vi "init_LiCor (moose's).vi"() -> ()   [LabVIEW 2010]
uses:
  <vilib>/Instr/_visa.llb/VISA Configure Serial Port (Instr).vi
panel:
  in  "String 3":string="(RS232(Poll Now))\\n "
  in  "String 2":string="(Display(BackLt\\s1))\\n "
  in  "String":string="(RS232(Sources (\"CO2B um/m\" \"H2OB mm/m\"  \"Integral\" \"Peak\" \"P kPa\" \"T C\" ))) "
  in  "Text_out 2":string
  in  "Text_out 1":string
  out "Text 2":string
  out "Text1":string
  out "VISA resource name 2":refnum<visa-resource-name>="ASRL2::INSTR"
  out "error out":errorcluster
  in  "init?":bool=TRUE
  in  "VISA resource name":refnum<visa-resource-name>="COM11"
  in  "error in":errorcluster
  in  "Quit?":bool=TRUE
  in  "Port Configuration":T1={"baud rate (9600)"=9600, "data bits (8)"=8, "parity (0:none)"=enum."None", "stop bits (10: 1 bit)"=10, "flow control (0:none)"=3, "timeout (10sec)"=10000, "termination char\n(0xA = '\\n' = LF) "=10, "Enable Termination\nChar (T)"=TRUE} {"termination char\n(0xA = '\\n' = LF)" format="%.0x"; "flow control (0:none)" items=["None", "XON/XOFF", "RTS/CTS", "XON/XOFF & RTS/CTS", "DTR/DSR", "XON/XOFF & DTR/DSR"]; "stop bits (10: 1 bit)" items=["1.0"=10, "1.5"=15, "2.0"=20]; "data bits (8)" min=5 max=8 step=1}
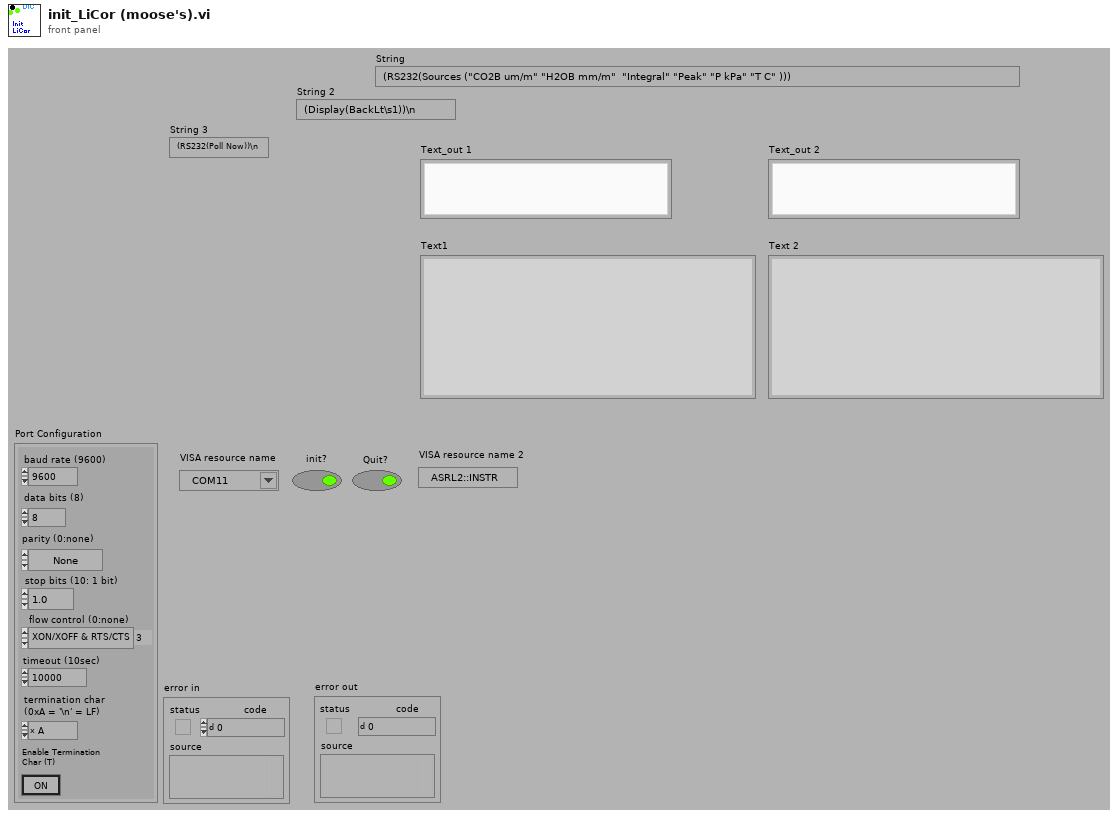
[diagram p1: front panel]
types:
  T1 = cluster{"baud rate (9600)":u32, "data bits (8)":u16, "parity (0:none)":enum16{"None", "Odd", "Even", "Mark", "Space"}, "stop bits (10: 1 bit)":u16, "flow control (0:none)":u16, "timeout (10sec)":u32, "termination char\n(0xA = '\\n' = LF) ":u8, "Enable Termination\nChar (T)":bool}
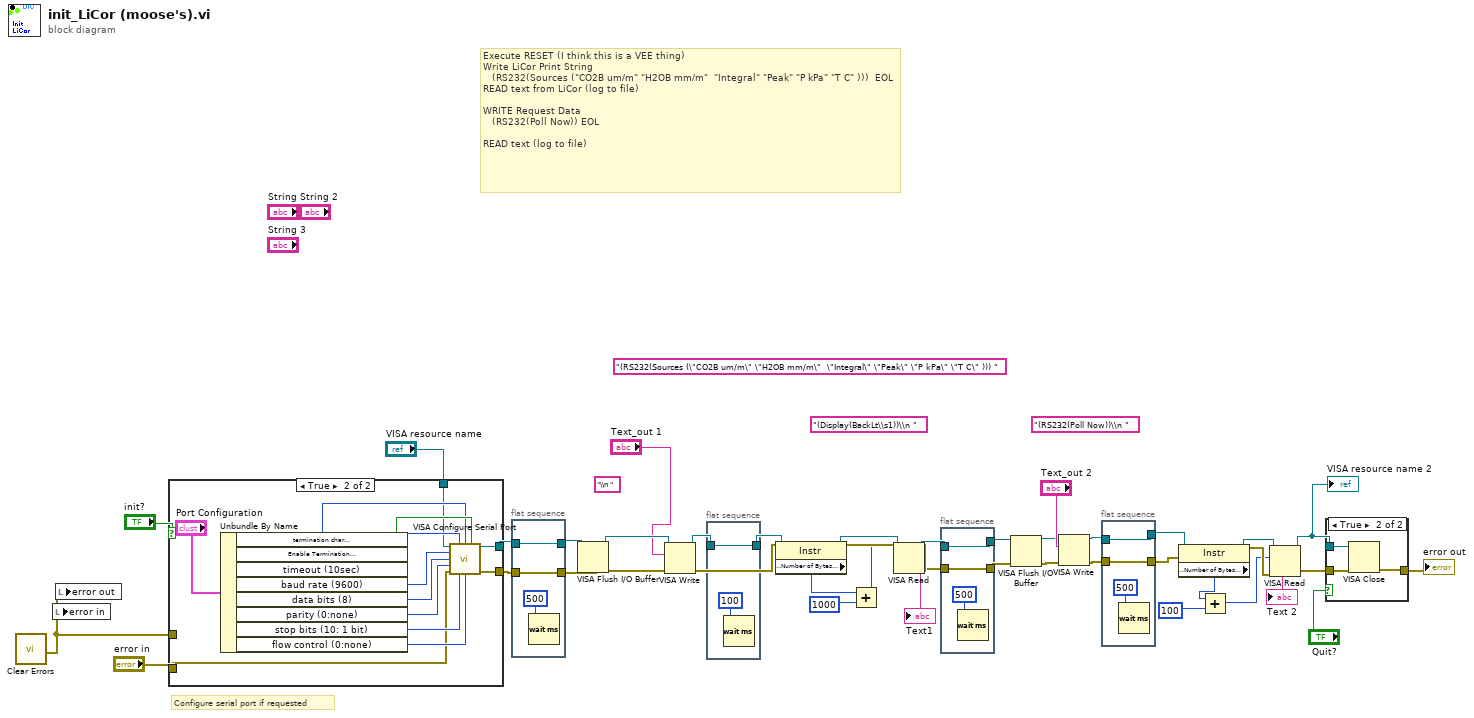
[diagram p0: block diagram]
diagram:
  (unwired) "\\n "
  (unwired) "(Display(BackLt\\s1))\\n "
  (unwired) "(RS232(Poll Now))\\n "
  (unwired) "(RS232(Sources (\"CO2B um/m\" \"H2OB mm/m\"  \"Integral\" \"Peak\" \"P kPa\" \"T C\" ))) "
  # "Configure serial port if requested"
  # "Execute RESET (I think this is a VEE thing)\nWrite LiCor Print String \n   (RS232(Sources (\"CO2B um/m\" \"H2OB mm/m\"  \"Integral\" \"Peak\" \"P kPa\" \"T C\" )))  EOL\nREAD text from LiCor (log to file)\n\nWRITE Request Data\n   (RS232(Poll Now)) EOL\n\nREAD text (log to file)"
  n1 = call <vilib>:"Clear Errors.vi"() -> ("error out"=w2:errorcluster)  [unwired: 7 in]
  n2 = local write "error in"(w2) -> ()
  n3 = local write "error out"(w2) -> ()
  n4 = case shown="True" "init?" {
    tunnel: [w42 w47] -> w21
    tunnel: [w43 w46] -> w19
    tunnel: "error in" -> [w43 w45]
    tunnel: "VISA resource name" -> [w42 w44]
    tunnel: w2 -> [_ _]
    frame False {
    }
    frame True {
      n5 = Unbundle By Name("Port Configuration") -> ("termination char\n(0xA = '\\n' = LF)"=w48:u8, "Enable Termination\nChar (T)"=w49:bool, "timeout (10sec)"=w50:u32, "baud rate (9600)"=w55:u32, "data bits (8)"=w54:u16, "parity (0:none)"=w53:enum16{"None", "Odd", "Even", "Mark", "Space"}, "stop bits (10: 1 bit)"=w52:u16, "flow control (0:none)"=w51:u16)
      n6 = call-poly "VISA Configure Serial Port"("VISA resource name"=w44, "timeout (10sec)"=w50, "termination char\n(0xA = '\\n' = LF)"=w48, "Enable Termination\nChar (T)"=w49, "baud rate (9600)"=w55, "data bits (8)"=w54, "parity (0:none)"=w53, "error in (no error)"=w45, "stop bits (10: 1 bit)"=w52, "flow control (0:none)"=w51) -> ("VISA resource name out"=w47:refnum<visa-resource-name>, "error out"=w46:errorcluster)  [unwired: 4 in]
    }
  }
  n7 = flat-sequence {
    tunnel: w21 -> [w59]
    tunnel: [w59] -> w20
    tunnel: w19 -> [w57]
    tunnel: [w57] -> w18
    frame #0 {
      n8 = Wait (ms)(milliseconds to wait=500) -> ()  [unwired: 1 out]
    }
  }
  n9 = VISA Flush I/O Buffer(VISA resource name=w20, error in (no error)=w18) -> (VISA resource name out=w37:refnum<visa-resource-name>, error out=w36:errorcluster)  [unwired: 1 in]
  n10 = VISA Write(VISA resource name=w37, write buffer="Text_out 1", error in (no error)=w36) -> (VISA resource name out=w26:refnum<visa-resource-name>, error out=w31:errorcluster)  [unwired: 1 out]
  n11 = flat-sequence {
    tunnel: w26 -> [w61]
    tunnel: [w61] -> w25
    frame #0 {
      n12 = Wait (ms)(milliseconds to wait=100) -> ()  [unwired: 1 out]
    }
  }
  n13 = property class="Instr"(reference=w25, error in=w31) -> (reference out=w30:refnum<visa-resource-name>, error out=w29:errorcluster, "Serial Settings:Number of Bytes at Serial Port"=w24:u32)
  n14 = Add(x=w24, y=1000) -> (x+y=w22:u32)
  n15 = VISA Read(VISA resource name=w30, byte count=w22, error in (no error)=w29) -> (VISA resource name out=w13:refnum<visa-resource-name>, read buffer=→"Text1":string, error out=w12:errorcluster)  [unwired: 1 out]
  n16 = flat-sequence {
    tunnel: [w62] -> w6
    tunnel: w12 -> [w63]
    tunnel: [w63] -> w7
    tunnel: w13 -> [w62]
    frame #0 {
      n17 = Wait (ms)(milliseconds to wait=500) -> ()  [unwired: 1 out]
    }
  }
  n18 = VISA Flush I/O Buffer(VISA resource name=w6, error in (no error)=w7) -> (VISA resource name out=w5:refnum<visa-resource-name>, error out=w4:errorcluster)  [unwired: 1 in]
  n19 = VISA Write(VISA resource name=w5, write buffer="Text_out 2", error in (no error)=w4) -> (VISA resource name out=w10:refnum<visa-resource-name>, error out=w9:errorcluster)  [unwired: 1 out]
  n20 = flat-sequence {
    tunnel: [w65] -> w11
    tunnel: w9 -> [w66]
    tunnel: [w66] -> w8
    tunnel: w10 -> [w65]
    frame #0 {
      n21 = Wait (ms)(milliseconds to wait=500) -> ()  [unwired: 1 out]
    }
  }
  n22 = property class="Instr"(reference=w11, error in=w8) -> (reference out=w28:refnum<visa-resource-name>, error out=w27:errorcluster, "Serial Settings:Number of Bytes at Serial Port"=w14:u32)
  n23 = Add(x=w14, y=100) -> (x+y=w15:u32)
  n24 = VISA Read(VISA resource name=w28, byte count=w15, error in (no error)=w27) -> (VISA resource name out=w33:refnum<visa-resource-name>, read buffer=→"Text 2":string, error out=w32:errorcluster)  [unwired: 1 out]
  "VISA resource name 2" <- w33
  n25 = case shown="True" "Quit?" {
    tunnel: w33 -> [_ w69]
    tunnel: w32 -> [w68 w71]
    tunnel: [w68 w70] -> w38
    frame False {
    }
    frame True {
      n26 = VISA Close(VISA resource name=w69, error in (no error)=w71) -> (error out=w70:errorcluster)
    }
  }
  "error out" <- w38
